vi "SelectMatchForPDF.vi"() -> (2 "Select Teams 2":u16(ring) items=["Q5", "Q13", "Q24", "Q31", "Q47", "Q59", "Q67", "Q72", "Q82", "All"])   [LabVIEW 2017]
panel:
  in  "OK":bool
  in  "Select Teams":u16(ring) items=["Q5", "Q13", "Q24", "Q31", "Q47", "Q59", "Q67", "Q72", "Q82", "All"]
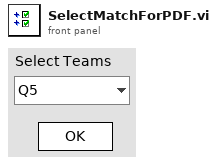
[diagram p1: front panel]
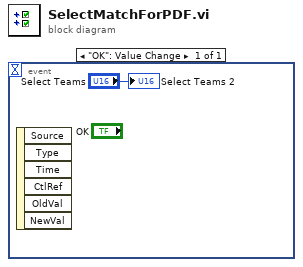
[diagram p0: block diagram]
diagram:
  n1 = event shown="[0] \"OK\": Value Change" {
    selector: _ -> [_]
    dyn-events: _ -> [_]
    timeout: _ -> [_]
    event "OK": Value Change {
      n2 = event-data() -> ()  [unwired: 1 in, 6 out]
      "Select Teams 2" <- "Select Teams"
    }
  }
